vi "_Set CellValue.vi"(8 "error in":errorcluster, 10 "CellValue in":refnum<k24>, 11 "Cell in":refnum<k24>) -> (0 "error out":errorcluster, 3 "Cell out":refnum<k24>)   [LabVIEW 2021, in "Open Xml.lvlib"]
uses:
  Open Xml.lvlib
  D:/git/Open-Xml-LabVIEW/dll/DocumentFormat.OpenXml.dll
  dll/DocumentFormat.OpenXml.dll
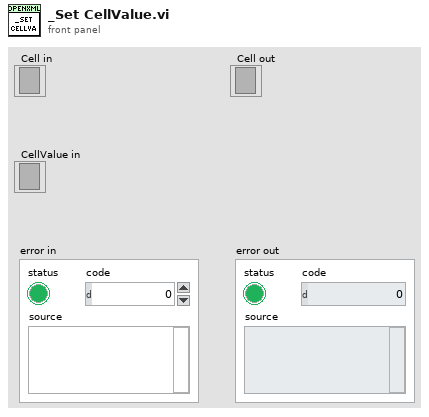
[diagram p1: front panel]
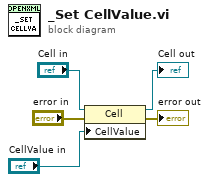
[diagram p0: block diagram]
diagram:
  n1 = property class="Cell"(reference="Cell in", error in="error in", "CellValue"="CellValue in") -> (reference out=→"Cell out":refnum<k24>, error out=→"error out":errorcluster)
